vi "MQTT_TCP_Open_Connection.vi"(6 "local port (0)":u16, 8 "error in (no error)":errorcluster, 9 "timeout ms (20000)":i32=20000, 10 "remote port or service name":u16=1883, 11 "address":string="green.daqloud.com") -> (0 "error out":errorcluster, 3 "connection ID":refnum<k5>)   [LabVIEW 2018, in "MQTT_Functions.lvlib"]
uses:
  MQTT_Functions.lvlib
panel:
  # "this is just a wrapper for the TCP Connect function\nadd or replace functionality as desired"
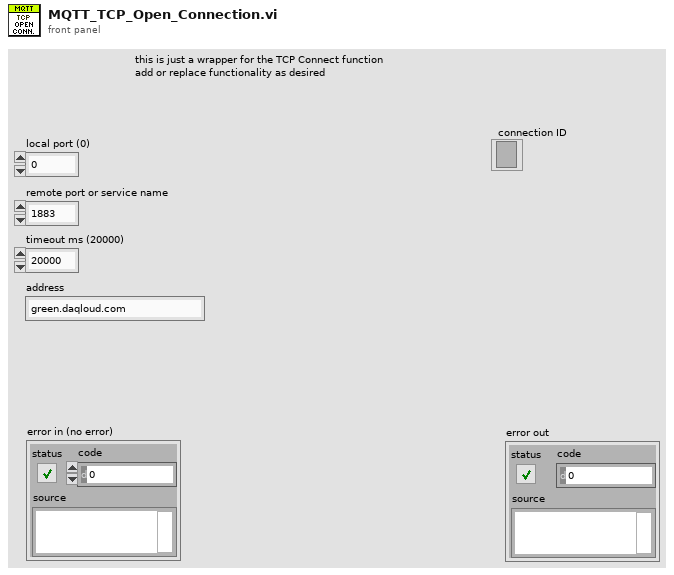
[diagram p1: front panel]
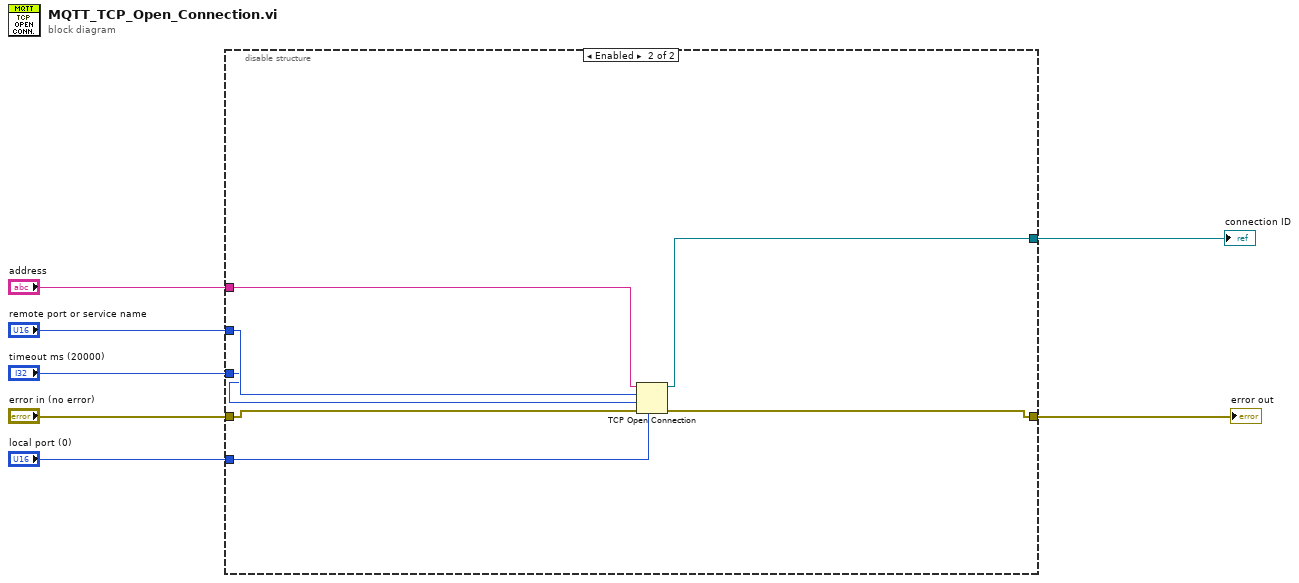
[diagram p0: block diagram]
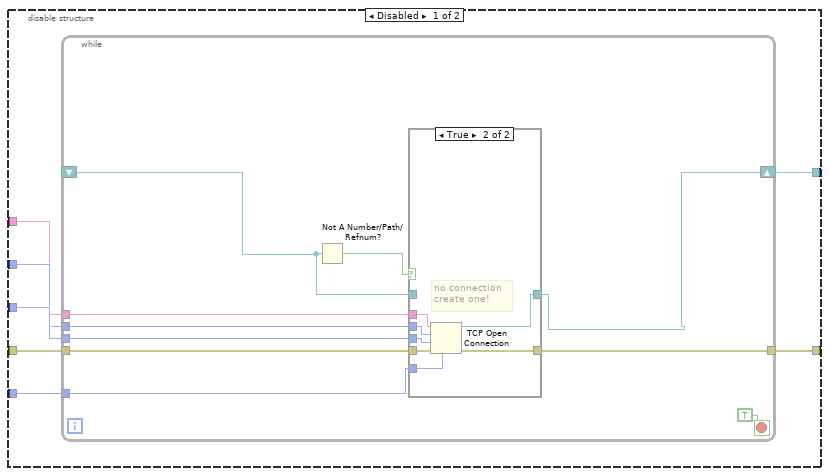
[diagram p2: hidden frame]
diagram:
  n1 = disable-structure shown="Enabled" {
    disable-tunnel: "local port (0)" -> [w14 w36]
    disable-tunnel: "error in (no error)" -> [w13 w37]
    disable-tunnel: "timeout ms (20000)" -> [w12 w38]
    disable-tunnel: "remote port or service name" -> [w11 w39]
    disable-tunnel: "address" -> [w10 w40]
    disable-tunnel: [w9 w34] -> w2
    disable-tunnel: [w8 w35] -> w1
    frame Disabled {
      n2 = while {
        tunnel: w14 -> [w24]
        tunnel: w13 -> [w23]
        tunnel: w12 -> [w22]
        tunnel: w11 -> [w18]
        tunnel: w10 -> [w21]
        tunnel: [w20] -> w9
        shift-right: [w15] -> w8
        shift-left: _ -> [w16]
        stop <- TRUE stop-if-true
        n3 = Not A Number/Path/Refnum?(number/path/refnum=w16) -> (NaN/Path/Refnum?=w17:bool)
        n4 = case shown="True" w17 {
          tunnel: w24 -> [_ w33]
          tunnel: w23 -> [w26 w32]
          tunnel: w22 -> [_ w31]
          tunnel: w18 -> [_ w30]
          tunnel: w21 -> [_ w29]
          tunnel: [w26 w28] -> w20
          tunnel: [w25 w27] -> w15
          tunnel: w16 -> [w25 _]
          frame False {
            # "retrieve last \nconnection ID"
          }
          frame True {
            # "no connection\ncreate one!"
            n5 = TCP Open Connection(address=w29, remote port or service name=w30, timeout ms (60000)=w31, local port=w33, error in (no error)=w32) -> (connection ID=w27:refnum<k5>, error out=w28:errorcluster)
          }
        }
      }
    }
    frame Enabled {
      n6 = TCP Open Connection(address=w40, remote port or service name=w39, timeout ms (60000)=w38, local port=w36, error in (no error)=w37) -> (connection ID=w35:refnum<k5>, error out=w34:errorcluster)
    }
  }
  "error out" <- w2
  "connection ID" <- w1
